vi "PUT (Buffer).vi"(6 "timeout":i32=10000, 7 "output file":path, 8 "error in":errorcluster, 9 "buffer":string, 10 "url":string, 11 "advanced-http-client in":refnum<class "advanced-http-client.lvclass">) -> (0 "error out":errorcluster, 2 "response out":refnum<class "response.lvclass">, 3 "advanced-http-client out":refnum<class "advanced-http-client.lvclass">)   [LabVIEW 2020, in "advanced-http-client.lvclass"]
uses:
  advanced-http-client.lvclass
  advanced-http-client.lvclass/advanced-http-client.ctl
  <vilib>/NI/Advanced HTTP Client/Session.lvclass
  response/response.lvclass
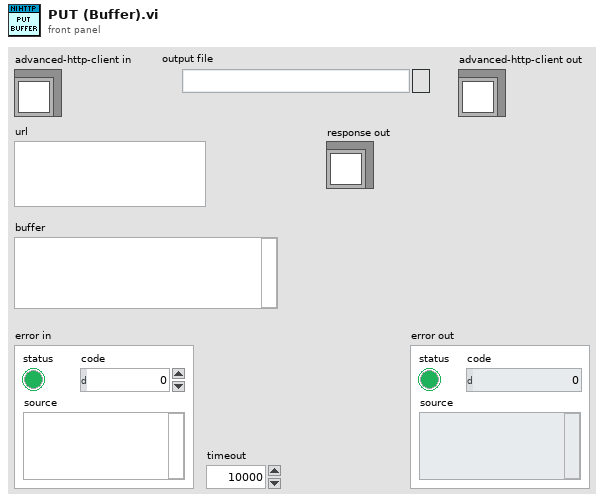
[diagram p1: front panel]
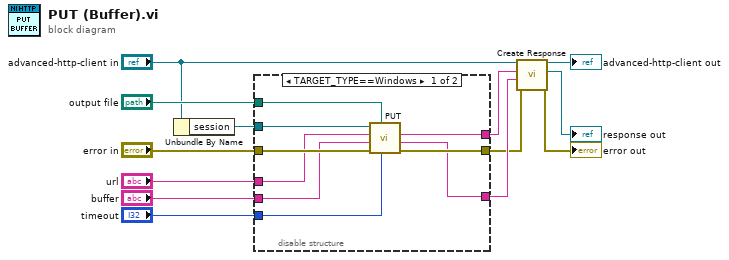
[diagram p0: block diagram]
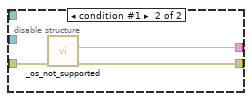
[diagram p2: hidden frame]
diagram:
  n1 = Unbundle By Name("advanced-http-client in") -> ("session"=w13:refnum<class "Session.lvclass">)
  n2 = disable-structure shown="TARGET_TYPE==Windows" {
    disable-tunnel: w13 -> [w22 _]
    disable-tunnel: "output file" -> [w21 _]
    disable-tunnel: "error in" -> [w20 w25]
    disable-tunnel: [w19 w24] -> w3
    disable-tunnel: "url" -> [w18 _]
    disable-tunnel: "buffer" -> [w17 _]
    disable-tunnel: "timeout" -> [w16 _]
    disable-tunnel: [w15 w23] -> w5
    disable-tunnel: [w14 _] -> w4
    frame condition #0 (active) {
      n3 = call-poly <vilib>:"PUT.vi"("timeout"=w16, "output file"=w21, "error in"=w20, "buffer"=w17, "url"=w18, "session in"=w22) -> ("error out"=w19:errorcluster, "body"=w14:string, "headers"=w15:string)  [unwired: 1 in, 2 out]
    }
    frame condition #1 {
      n4 = call "_os_not_supported.vi"("error in (no error)"=w25) -> ("error out"=w24:errorcluster, "headers"=w23:string)  [unwired: 9 in]
    }
  }
  n5 = call-dynamic "Create Response.vi"("error in (no error)"=w3, "body"=w4, "headers"=w5, "http-client"="advanced-http-client in") -> ("error out"=→"error out":errorcluster, "response out"=→"response out":refnum<class "response.lvclass">, "http-client out"=→"advanced-http-client out":refnum<class "advanced-http-client.lvclass">)  [unwired: 5 in]
